vi "SMR_LabVIEW_V6.75.vi"() -> ()   [LabVIEW 2025]
uses:
  <vilib>/DAQmx/read.llb/DAQmx Read (Analog 1D DBL NChan 1Samp).vi
  <vilib>/DAQmx/create/channels.llb/DAQmx Create Channel (AI-Temperature-Thermocouple).vi
  <vilib>/DAQmx/create/channels.llb/DAQmx Create Channel (AI-Voltage-Basic).vi
  <vilib>/DAQmx/miscellaneous.llb/DAQmx Fill In Error Info.vi
panel:
  out "Rate Window Ready":bool
  out "Steady State":bool
  in  "Steady State Threshold (deg C/min)":dbl=0.5
  out "Temp Change Rate (deg C/min)":dbl
  in  "Voltage Limit (V)":dbl=10.0
  in  "Temperature Limit (C)":dbl=50.0
  in  "Pressure Limit (psi)":dbl=15.0
  out "Max Voltage":bool
  out "Max Temperature":bool
  out "Max Pressure":bool
  out "Current Run Folder":path
  in  "Log Root Folder":path=path "C:/Users/LocalUser/Documents/GitHub/thermal-loop/resources/v0.1.1/data/001"
  out "Heat Exchanger Pressure History":dbl(graph)
  out "Main Loop Pressure History":T1(graph)
  out "Heat Exchanger Temperature History":cluster{"Waveform":dbl, "Waveform":dbl}(graph)
  out "Main Loop Temeperature History":T2(graph)
  out "Overall Avg Pressure (psi)":dbl
  out "Heat Exchanger Pressure P6 (psi)":dbl
  out "Main Loop Avg Pressure (psi)":dbl
  out "Heat Exchanger Avg Temp (deg C)":dbl
  out "Main Loop Avg Temp (deg C)":dbl
  out "Raw NI9201 \nVoltage Display":T3
  out "Temperature Display":T4
  out "Pressure Display":T5
  in  "Flow Offset Correction (GPM)":dbl=-0.3
  out "Flow History":dbl(graph)
  out "Overall Pressure History":T6(graph)
  out "Overall Temperature History":T7(graph)
  out "Max Loop Pressure (psi)":dbl
  out "Overall Avg Temp (deg C)":dbl
  out "Max Loop Temp (deg C)":dbl
  out "Heat Exchanger Flow (GPM)":dbl
  in  "Loop Period (ms)":dbl=1000.0
  in  "Stop":bool
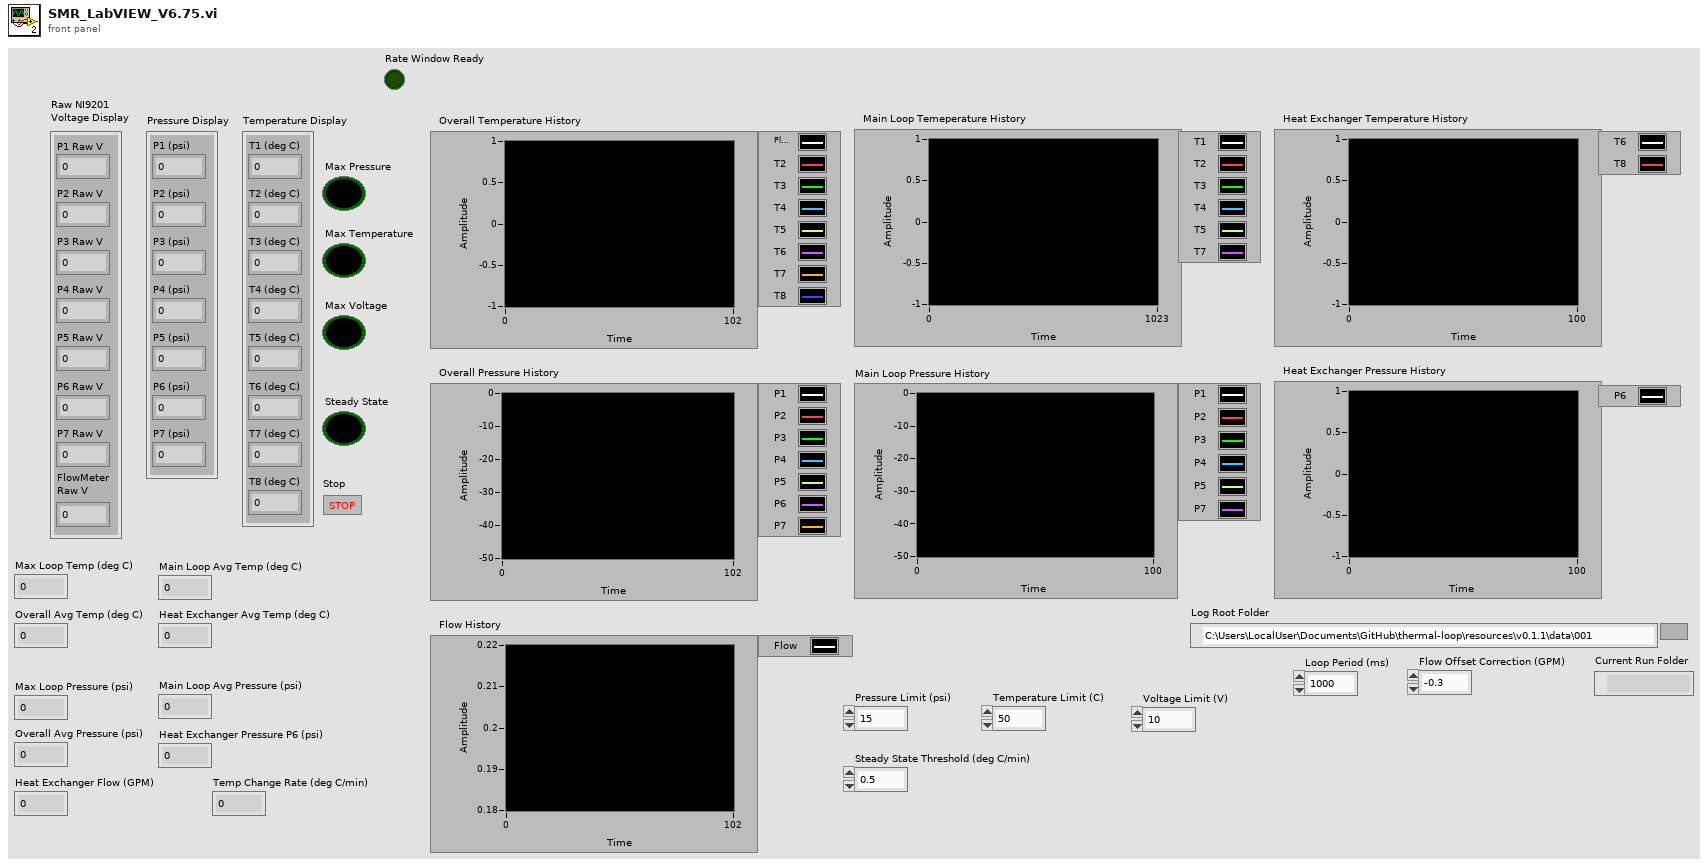
[diagram p1: front panel]
types:
  T1 = cluster{"P1":dbl, "P2":dbl, "P3":dbl, "P4":dbl, "P5":dbl, "P7":dbl}
  T2 = cluster{"Waveform":dbl, "Waveform":dbl, "Waveform":dbl, "Waveform":dbl, "Waveform":dbl, "Waveform":dbl}
  T3 = cluster{"P1 Raw V":dbl, "P2 Raw V":dbl, "P3 Raw V":dbl, "P4 Raw V":dbl, "P5 Raw V":dbl, "P6 Raw V":dbl, "P7 Raw V":dbl, "FlowMeter\nRaw V":dbl}
  T4 = cluster{"T1 (deg C)":dbl, "T2 (deg C)":dbl, "T3 (deg C)":dbl, "T4 (deg C)":dbl, "T5 (deg C)":dbl, "T6 (deg C)":dbl, "T7 (deg C)":dbl, "T8 (deg C)":dbl}
  T5 = cluster{"P1 (psi)":dbl, "P2 (psi)":dbl, "P3 (psi)":dbl, "P4 (psi)":dbl, "P5 (psi)":dbl, "P6 (psi)":dbl, "P7 (psi)":dbl}
  T6 = cluster{"P1":dbl, "P2":dbl, "P3":dbl, "P4":dbl, "P5":dbl, "P6":dbl, "P7":dbl}
  T7 = cluster{"Waveform":dbl, "Waveform":dbl, "Waveform":dbl, "Waveform":dbl, "Waveform":dbl, "Waveform":dbl, "Waveform":dbl, "Waveform":dbl}
  T8 = enum16{"open", "replace", "create", "open or create", "replace or create", "replace or create with confirmation"}
  T9 = cluster{"P1":dbl, "P2":dbl, "P3":dbl, "P4":dbl, "P5":dbl, "P6":dbl, "P7":dbl, "Flow":dbl}
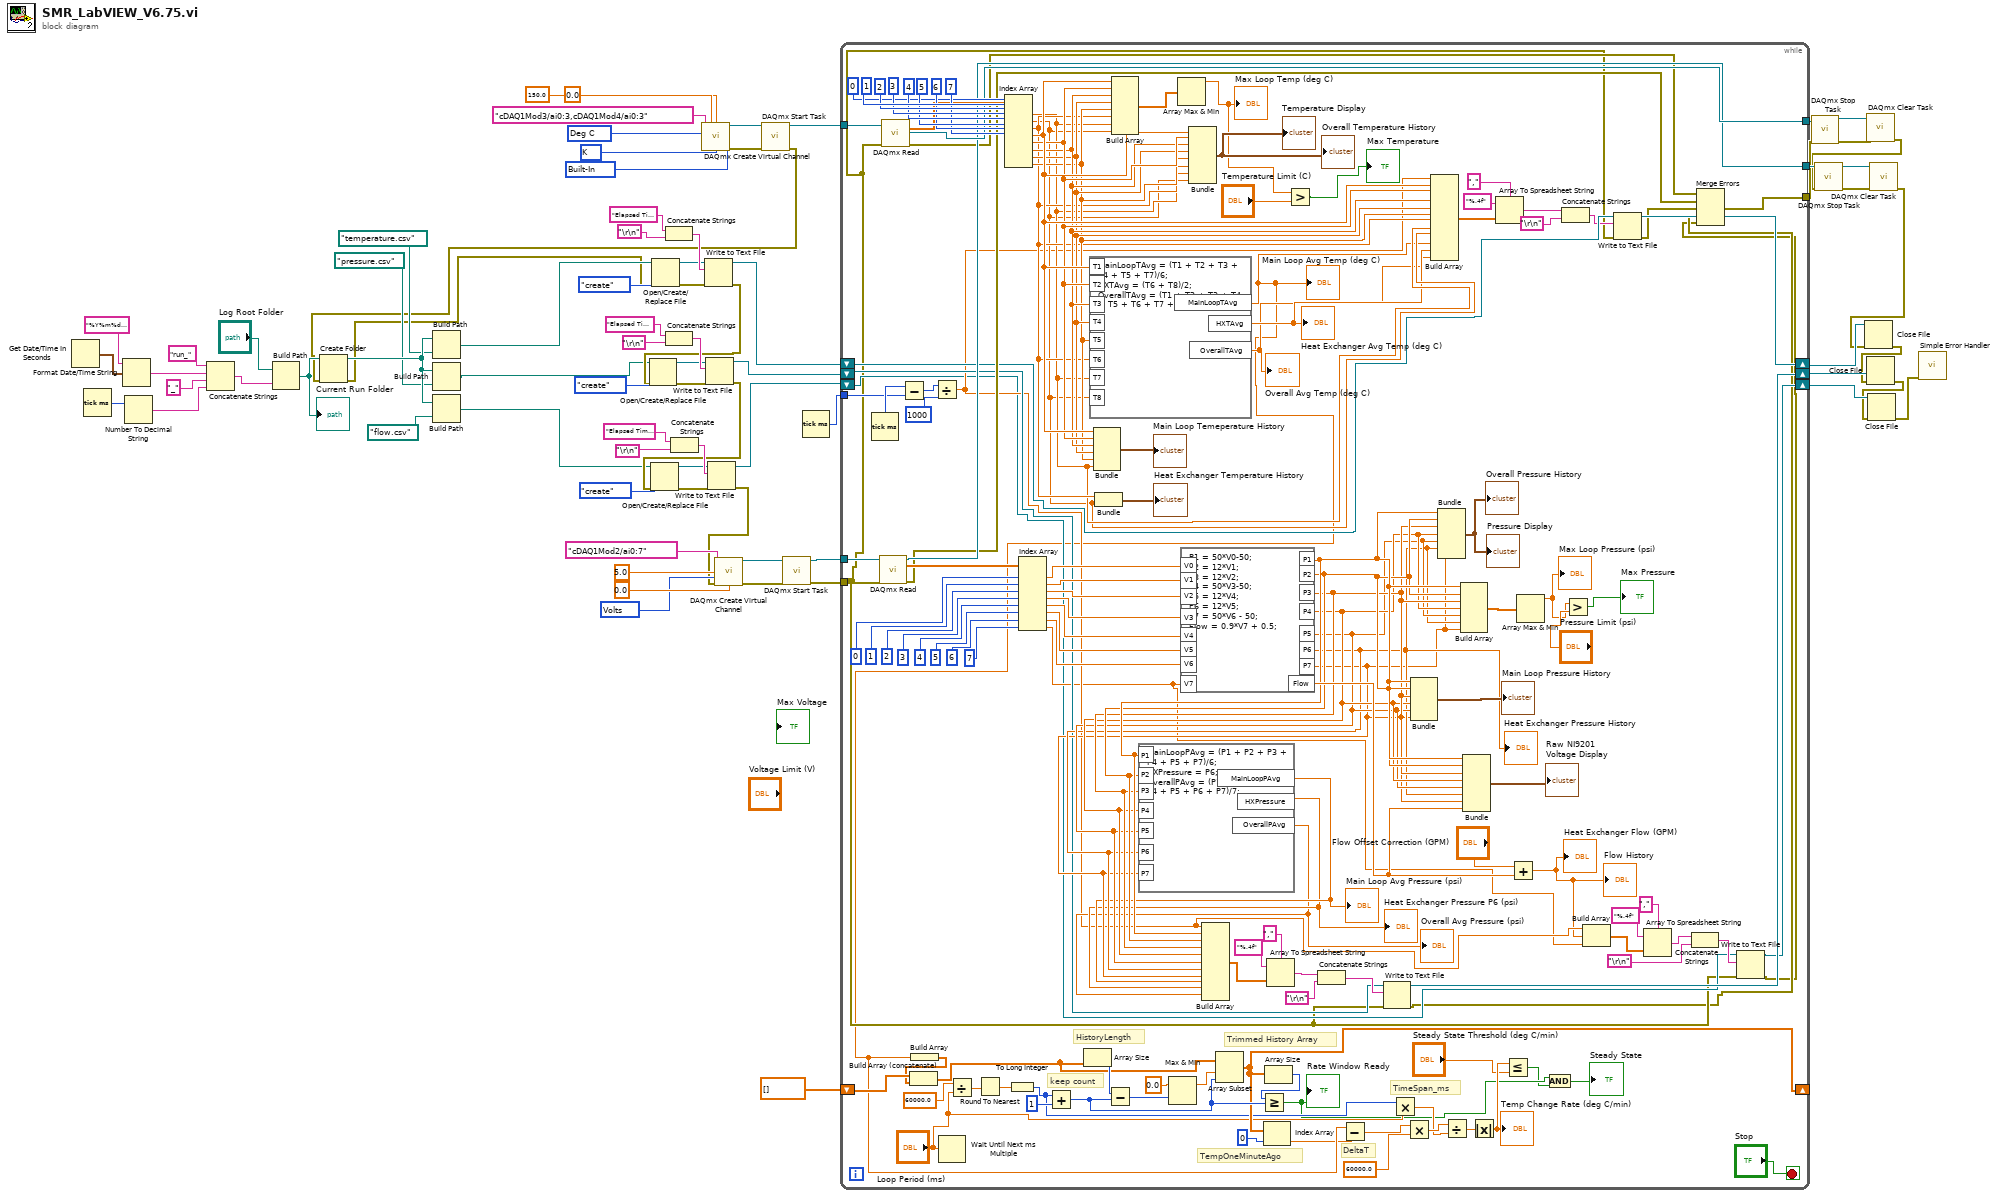
[diagram p0: block diagram]
diagram:
  w65 = 10200 items=["Built-In"=10200, "Constant Value"=10116, "Channel"=10113] ("cjc source")
  w66 = 10073 items=["J"=10072, "K"=10073, "N"=10077, "R"=10082, "S"=10085, "T"=10086, "B"=10047, "E"=10055] ("thermocouple type")
  w67 = 10143 items=["Deg C"=10143, "Deg F"=10144, "Kelvins"=10325, "Deg R"=10145, "From Custom Scale"=10065] ("units")
  w74 = 10348 items=["Volts"=10348, "From Custom Scale"=10065] ("units")
  n1 = Get Date/Time In Seconds() -> (seconds since 1Jan1904=w20:timestamp)
  n2 = Tick Count (ms)() -> (millisecond timer value=w18:u32)
  n3 = Format Date/Time String(time format string (%c)="%Y%m%d_%H%M%S", seconds (now)=w20) -> (date/time string=w15:string)  [unwired: 1 in]
  n4 = Number To Decimal String(number=w18) -> (decimal integer string=w16:string)  [unwired: 1 in]
  n5 = Concatenate Strings("run_" ("string"), w15, "_" ("string"), w16) -> (w12:string)
  n6 = Build Path(base path="Log Root Folder", name or relative path=w12) -> (appended path=w11:path)
  "Current Run Folder" <- w11
  n7 = Concatenate Strings("Elapsed Time (s),T1 (deg C),T2 (deg C),T3 (deg C),T4 (deg C),T5 (deg C),T6 (deg C),T7 (deg C),T8 (deg C),Main Loop Avg Temp (deg C),HX Avg Temp (deg C),Overall Avg Temp (deg C)", "\r\n") -> (w47:string)
  n8 = Concatenate Strings("Elapsed Time (s),P1 (psi),P2 (psi),P3 (psi),P4 (psi),P5 (psi),P6 (psi),P7 (psi),Main Loop Avg Pressure (psi),HX Pressure (psi),Overall Avg Pressure (psi)", "\r\n") -> (w45:string)
  n9 = Concatenate Strings("Elapsed Time (s),Heat Exchanger Flow (GPM),Flow Raw Voltage (V)", "\r\n") -> (w41:string)
  n10 = call-poly <vilib>:"DAQmx Create Virtual Channel.vi"("maximum value"=150.0, "minimum value"=0.0, "physical channels"=tag "cDAQ1Mod3/ai0:3,cDAQ1Mod4/ai0:3", "cjc source"=w65, "units"=w67, "thermocouple type"=w66) -> ("task out"=w64:refnum<k21>, "error out"=w63:errorcluster)  [unwired: 8 in]
  n11 = call <vilib>:"DAQmx Start Task.vi"("task/channels in"=w64, "error in"=w63) -> ("task out"=w62:refnum<k21>, "error out"=w3:errorcluster)  [unwired: 12 in]
  n12 = Create Folder(path (use dialog)=w11, error in=w3) -> (created path=w10:path, error out=w2:errorcluster)  [unwired: 1 in, 1 out]
  n13 = Build Path(base path=w10, name or relative path=path "temperature.csv") -> (appended path=w9:path)
  n14 = Build Path(base path=w10, name or relative path=path "pressure.csv") -> (appended path=w8:path)
  n15 = Build Path(base path=w10, name or relative path=path "flow.csv") -> (appended path=w7:path)
  n16 = Open/Create/Replace File(file path (use dialog)=w9, error in=w2, operation (0:open)=T8."create") -> (refnum out=w46:refnum<file>, error out=w30:errorcluster)  [unwired: 3 in, 1 out]
  n17 = Write to Text File(file (use dialog)=w46, text=w47, error in=w30) -> (refnum out=w37:refnum<file>, error out=w29:errorcluster)  [unwired: 1 in, 1 out]
  n18 = Open/Create/Replace File(file path (use dialog)=w8, error in=w29, operation (0:open)=T8."create") -> (refnum out=w44:refnum<file>, error out=w28:errorcluster)  [unwired: 3 in, 1 out]
  n19 = Write to Text File(file (use dialog)=w44, text=w45, error in=w28) -> (refnum out=w36:refnum<file>, error out=w27:errorcluster)  [unwired: 1 in, 1 out]
  n20 = Open/Create/Replace File(file path (use dialog)=w7, error in=w27, operation (0:open)=T8."create") -> (refnum out=w40:refnum<file>, error out=w26:errorcluster)  [unwired: 3 in, 1 out]
  n21 = Write to Text File(file (use dialog)=w40, text=w41, error in=w26) -> (refnum out=w35:refnum<file>, error out=w25:errorcluster)  [unwired: 1 in, 1 out]
  n22 = call-poly <vilib>:"DAQmx Create Virtual Channel.vi"("maximum value"=5.0, "minimum value"=0.0, "physical channels"=tag "cDAQ1Mod2/ai0:7", "units"=w74, "error in"=w25) -> ("task out"=w73:refnum<k21>, "error out"=w72:errorcluster)  [unwired: 9 in]
  n23 = call <vilib>:"DAQmx Start Task.vi"("task/channels in"=w73, "error in"=w72) -> ("task out"=w71:refnum<k21>, "error out"=w60:errorcluster)  [unwired: 12 in]
  n24 = Tick Count (ms)() -> (millisecond timer value=w34:u32)
  n25 = while {
    tunnel: w71 -> [w208]
    tunnel: w62 -> [w182]
    tunnel: [w172] -> w61
    tunnel: w60 -> [w116]
    tunnel: [w171] -> w59
    tunnel: [w168] -> w58
    shift-right: [w147] -> w33
    shift-left: w37 -> [w148]
    shift-right: [w128] -> w32
    shift-left: w36 -> [w129]
    shift-right: [w117] -> w31
    shift-left: w35 -> [w118]
    tunnel: w34 -> [w166]
    shift-right: [w93] -> _
    shift-left: dbl[] [] -> [w106]
    stop <- "Stop" stop-if-true
    # "TimeSpan_ms"
    # "DeltaT"
    # "TempOneMinuteAgo"
    # "Trimmed History Array"
    # "HistoryLength"
    # "keep count"
    n26 = Tick Count (ms)() -> (millisecond timer value=w167:u32)
    n27 = call-poly <vilib>:"DAQmx Read.vi"("task/channels in"=w208, "error in"=w116) -> ("task out"=w171:refnum<k21>, "data"=w199:dbl[], "error out"=w169:errorcluster)  [unwired: 11 in]
    n28 = call-poly <vilib>:"DAQmx Read.vi"("task/channels in"=w182, "error in"=w116) -> ("task out"=w172:refnum<k21>, "data"=w173:dbl[], "error out"=w170:errorcluster)  [unwired: 11 in]
    n29 = Subtract(x=w167, y=w166) -> (x-y=w165:u32)
    n30 = Divide(x=w165, y=u32 1000) -> (x/y=w127:dbl)
    n31 = Wait Until Next ms Multiple(millisecond multiple="Loop Period (ms)") -> ()  [unwired: 1 out]
    n32 = Divide(x=60000.0, y="Loop Period (ms)") -> (x/y=w103:dbl)
    n33 = Round To Nearest(number=w103) -> (nearest integer value=w102:dbl)
    n34 = Index Array(array=w173, index #1=0 ("index"), index #2=1 ("index"), index #3=2 ("index"), index #4=3 ("index"), index #5=4 ("index"), index #6=5 ("index"), index #7=6 ("index"), index #8=7 ("index")) -> (element #1=w157:dbl, element #2=w156:dbl, element #3=w158:dbl, element #4=w163:dbl, element #5=w162:dbl, element #6=w161:dbl, element #7=w160:dbl, element #8=w159:dbl)
    n35 = To Long Integer(number=w102) -> (32bit integer=w89:i32)
    n36 = Index Array(array=w199, index #1=0 ("index"), index #2=1 ("index"), index #3=2 ("index"), index #4=3 ("index"), index #5=4 ("index"), index #6=5 ("index"), index #7=6 ("index"), index #8=7 ("index")) -> (element #1=w198:dbl, element #2=w197:dbl, element #3=w196:dbl, element #4=w195:dbl, element #5=w194:dbl, element #6=w193:dbl, element #7=w192:dbl, element #8=w125:dbl)
    n37 = Add(x=w89, y=1) -> (x+y=w95:i32)
    n38 = formula code="MainLoopTAvg = (T1 + T2 + T3 + T4 + T5 + T7)/6;\nHXTAvg = (T6 + T8)/2;\nOverallTAvg = (T1 + T2 + T3 + T4 + T5 + T6 + T7 + T8)/8;"("T1"=w163, "T2"=w162, "T3"=w161, "T4"=w160, "T5"=w159, "T6"=w158, "T7"=w157, "T8"=w156) -> ("MainLoopTAvg"=w91:dbl, "HXTAvg"=w155:dbl, "OverallTAvg"=w154:dbl)
    "Overall Avg Temp (deg C)" <- w154
    "Main Loop Avg Temp (deg C)" <- w91
    "Heat Exchanger Avg Temp (deg C)" <- w155
    n39 = Build Array(w91) -> (w105:dbl[])
    n40 = Build Array (concatenate)(w106, w105) -> (w97:dbl[])
    n41 = Array Size(array=w97) -> (size(s)=w100:i32)
    n42 = Bundle("Waveform"=w163, "Waveform"=w162, "Waveform"=w161, "Waveform"=w160, "Waveform"=w159, "Waveform"=w157) -> (→"Main Loop Temeperature History":T2)  [unwired: 1 in]
    n43 = Bundle("Waveform"=w158, "Waveform"=w156) -> (→"Heat Exchanger Temperature History":cluster{"Waveform":dbl, "Waveform":dbl})  [unwired: 1 in]
    n44 = Subtract(x=w100, y=w95) -> (x-y=w98:i32)
    n45 = Build Array(w163, w162, w161, w160, w159, w158, w157, w156) -> (w209:dbl[])
    n46 = Max & Min(x=0.0, y=w98) -> (max(x,y)=w96:dbl)  [unwired: 1 out]
    n47 = Array Max & Min(array=w209) -> (max value=w109:dbl)  [unwired: 3 out]
    "Max Loop Temp (deg C)" <- w109
    n48 = formula code="P1 = 50*V0-50;\nP2 = 12*V1;\nP3 = 12*V2;\nP4 = 50*V3-50;\nP5 = 12*V4;\nP6 = 12*V5; \nP7 = 50*V6 - 50;\nFlow = 0.9*V7 + 0.5;"("V0"=w198, "V1"=w197, "V2"=w196, "V3"=w195, "V4"=w194, "V5"=w193, "V6"=w192, "V7"=w125) -> ("P1"=w146:dbl, "P2"=w145:dbl, "P3"=w144:dbl, "P4"=w143:dbl, "P5"=w142:dbl, "P6"=w141:dbl, "P7"=w140:dbl, "Flow"=w187:dbl)
    "Heat Exchanger Pressure History" <- w141
    n49 = formula code="MainLoopPAvg = (P1 + P2 + P3 + P4 + P5 + P7)/6;\nHXPressure = P6;\nOverallPAvg = (P1 + P2 + P3 + P4 + P5 + P6 + P7)/7;"("P1"=w146, "P2"=w145, "P3"=w144, "P4"=w143, "P5"=w142, "P6"=w141, "P7"=w140) -> ("MainLoopPAvg"=w139:dbl, "HXPressure"=w138:dbl, "OverallPAvg"=w137:dbl)
    "Overall Avg Pressure (psi)" <- w137
    "Heat Exchanger Pressure P6 (psi)" <- w138
    "Main Loop Avg Pressure (psi)" <- w139
    n50 = Bundle("Waveform"=w163, "Waveform"=w162, "Waveform"=w161, "Waveform"=w160, "Waveform"=w159, "Waveform"=w158, "Waveform"=w157, "Waveform"=w156) -> (→"Overall Temperature History" →"Temperature Display":T7)  [unwired: 1 in]
    n51 = Build Array(w127, w146, w145, w144, w143, w142, w141, w140, w139, w138, w137) -> (w136:dbl[])
    n52 = Array Subset(array=w97, index=w96, length=w95) -> (w93:dbl[])
    n53 = Index Array(array=w93, index=0) -> (element=w90:dbl)
    n54 = Array Size(array=w93) -> (size(s)=w94:i32)
    n55 = Greater Or Equal?(x=w94, y=w95) -> (x >= y?=w80:bool)
    "Rate Window Ready" <- w80
    n56 = Array To Spreadsheet String(delimiter (Tab)=",", array=w136, 3:"%.4f" ("format string")) -> (spreadsheet string=w132:string)
    n57 = Greater?(x=w109, y="Temperature Limit (C)") -> (0:→"Max Temperature":bool)
    n58 = Concatenate Strings(w132, "\r\n") -> (w130:string)
    n59 = Subtract(x=w91, y=w90) -> (x-y=w87:dbl)
    n60 = Write to Text File(file (use dialog)=w129, text=w130, error in=w116) -> (refnum out=w128:refnum<file>, error out=w114:errorcluster)  [unwired: 1 in, 1 out]
    n61 = Multiply(x=w89, y="Loop Period (ms)") -> (x*y=w84:dbl)
    n62 = Multiply(x=w87, y=60000.0) -> (x*y=w85:dbl)
    n63 = Bundle("P1"=w146, "P2"=w145, "P3"=w144, "P4"=w143, "P5"=w142, "P7"=w140) -> (→"Main Loop Pressure History":T1)  [unwired: 1 in]
    n64 = Build Array(w127, w163, w162, w161, w160, w159, w158, w157, w156, w91, w155, w154) -> (w153:dbl[])
    n65 = Bundle("P1"=w146, "P2"=w145, "P3"=w144, "P4"=w143, "P5"=w142, "P6"=w141, "P7"=w140) -> (→"Overall Pressure History" →"Pressure Display":T6)  [unwired: 1 in]
    n66 = Divide(x=w85, y=w84) -> (x/y=w83:dbl)
    n67 = Build Array(w146, w145, w144, w143, w142, w141, w140) -> (w190:dbl[])
    n68 = Bundle("P1"=w146, "P2"=w145, "P3"=w144, "P4"=w143, "P5"=w142, "P6"=w141, "P7"=w140, "Flow"=w187) -> (→"Raw NI9201 \nVoltage Display":T9)  [unwired: 1 in]
    n69 = Absolute Value(x=w83) -> (abs(x)=w82:dbl)
    "Temp Change Rate (deg C/min)" <- w82
    n70 = Array To Spreadsheet String(delimiter (Tab)=",", array=w153, 3:"%.4f" ("format string")) -> (spreadsheet string=w150:string)
    n71 = Less Or Equal?(x=w82, y="Steady State Threshold (deg C/min)") -> (x <= y?=w79:bool)
    n72 = Add(x="Flow Offset Correction (GPM)", y=w187) -> (x+y=w126:dbl)
    "Heat Exchanger Flow (GPM)" <- w126
    "Flow History" <- w126
    n73 = Array Max & Min(array=w190) -> (max value=w111:dbl)  [unwired: 3 out]
    "Max Loop Pressure (psi)" <- w111
    n74 = And(x=w80, y=w79) -> (x .and. y?=→"Steady State":bool)
    n75 = Concatenate Strings(w150, "\r\n") -> (w133:string)
    n76 = Greater?(x=w111, y="Pressure Limit (psi)") -> (0:→"Max Pressure":bool)
    n77 = Build Array(w127, w126, w125) -> (w124:dbl[])
    n78 = Write to Text File(file (use dialog)=w148, text=w133, error in=w116) -> (refnum out=w147:refnum<file>, error out=w115:errorcluster)  [unwired: 1 in, 1 out]
    n79 = Array To Spreadsheet String(delimiter (Tab)=",", array=w124, 3:"%.4f" ("format string")) -> (spreadsheet string=w120:string)
    n80 = Concatenate Strings(w120, "\r\n") -> (w119:string)
    n81 = Write to Text File(file (use dialog)=w118, text=w119, error in=w116) -> (refnum out=w117:refnum<file>, error out=w113:errorcluster)  [unwired: 1 in, 1 out]
    n82 = Merge Errors(w170, w169, w115, w114, w113) -> (w168:errorcluster)
  }
  n83 = call <vilib>:"DAQmx Stop Task.vi"("task/channels in"=w61, "error in"=w58) -> ("task out"=w57:refnum<k21>, "error out"=w55:errorcluster)  [unwired: 12 in]
  n84 = call <vilib>:"DAQmx Clear Task.vi"("task in"=w57, "error in"=w55) -> ("error out"=w54:errorcluster)  [unwired: 13 in]
  n85 = call <vilib>:"DAQmx Stop Task.vi"("task/channels in"=w59, "error in"=w54) -> ("task out"=w56:refnum<k21>, "error out"=w53:errorcluster)  [unwired: 12 in]
  n86 = call <vilib>:"DAQmx Clear Task.vi"("task in"=w56, "error in"=w53) -> ("error out"=w24:errorcluster)  [unwired: 13 in]
  n87 = Close File(refnum=w33, error in=w24) -> (error out=w23:errorcluster)  [unwired: 1 out]
  n88 = Close File(refnum=w32, error in=w23) -> (error out=w22:errorcluster)  [unwired: 1 out]
  n89 = Close File(refnum=w31, error in=w22) -> (error out=w21:errorcluster)  [unwired: 1 out]
  n90 = call <vilib>:"Simple Error Handler.vi"("error in (no error)"=w21) -> ()  [unwired: 4 in, 5 out]
